vi "dfd_Symmetric or not.vi"(10 "Coef":dbl[](array[numeric])) -> (2 "Symmetric?":bool)   [LabVIEW 2017, in "NI_DigFilter_Process.lvlib"]
uses:
  <vilib>/addons/Digital Filter Design/NI_DigFilter_Process.lvlib
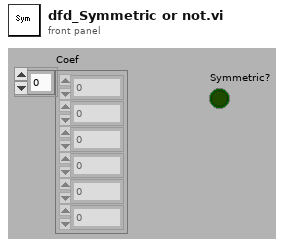
[diagram p1: front panel]
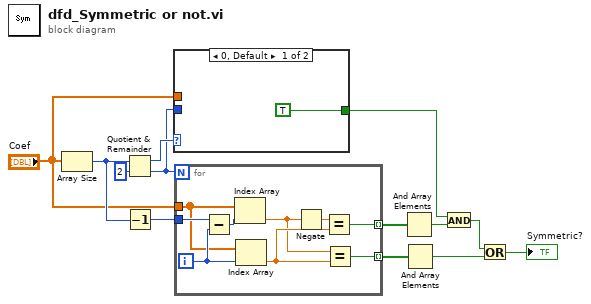
[diagram p0: block diagram]
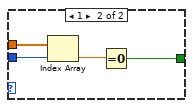
[diagram p2: hidden frame]
diagram:
  n1 = Array Size(array="Coef") -> (size(s)=w11:i32)
  n2 = Quotient & Remainder(x=w11, y=2) -> (x-y*floor(x/y)=w8:i32, floor(x/y)=w7:i32)
  n3 = Decrement(x=w11) -> (x-1=w13:i32)
  n4 = case shown="0, Default" w8 {
    tunnel: w7 -> [_ w18]
    tunnel: "Coef" -> [_ w17]
    tunnel: [TRUE w15] -> w3
    frame 0, Default {
    }
    frame 1 {
      n5 = Index Array(array=w17, index=w18) -> (element=w16:dbl)
      n6 = Equal To 0?(x=w16) -> (x = 0?=w15:bool)
    }
  }
  n7 = for {
    N: w7 -> [_]
    tunnel: w13 -> [w27]
    tunnel: "Coef" -> [w24]
    tunnel: [w23] -> w10 mode=indexing
    tunnel: [w22] -> w9 mode=indexing
    i -> [w26]
    n8 = Subtract(x=w27, y=w26) -> (x-y=w25:i32)
    n9 = Index Array(array=w24, index=w25) -> (element=w20:dbl)
    n10 = Index Array(array=w24, index=w26) -> (element=w21:dbl)
    n11 = Negate(x=w20) -> (-x=w19:dbl)
    n12 = Equal?(x=w19, y=w21) -> (x = y?=w23:bool)
    n13 = Equal?(x=w20, y=w21) -> (x = y?=w22:bool)
  }
  n14 = And Array Elements(Boolean array=w10) -> (logical AND=w4:bool)
  n15 = And Array Elements(Boolean array=w9) -> (logical AND=w5:bool)
  n16 = And(x=w3, y=w4) -> (x .and. y?=w2:bool)
  n17 = Or(x=w2, y=w5) -> (x .or. y?=→"Symmetric?":bool)
